vi "Set Application Error.vi"(4 "Time Stamp":timestamp, 5 "Error Name":string, 6 "Error Message":string, 7 "Error Scope":string, 8 "Error In":errorcluster, 9 "Call Chain":string[](array[string]), 10 "Log Error?":bool, 11 "Error Source":string) -> (0 "Error Out":errorcluster)   [LabVIEW 2016, in "Stream Error.lvlib" / "Application Error.lvclass"]
doc: "--\nCopyright © 2017 Composed SystemsI All rights reserved.\n\nAuthor: Jon McBee <jon.mcbee@composed.io>\n\nThis library is provided \"AS IS\" ,WITHOUT WARRANTIES OR\nCONDITIONS OF ANY KIND, either express or implied.\n\nComposed Systems -- composed.io\n\nStream 0.0.1.1\nJon McBee - Composed Systems\nCopyright (c) 2017, Composed Systems"
uses:
  <userlib>/Composed Systems/Stream/Error/Classes/Application Error/Application Error.lvclass
  <userlib>/Composed Systems/Stream/Error/Classes/Error Interface/Error Interface.lvclass
  <userlib>/Composed Systems/Stream/Error/Classes/Error Interface/Error Interface.lvclass/Error Interface.ctl
  <userlib>/Composed Systems/Stream/Log/Application Log/Log Level.ctl
  <userlib>/Composed Systems/Stream/Log/Global Application Log/Global Application Log.lvclass
  <userlib>/Composed Systems/Stream/Log/Application Log/Application Log.lvclass
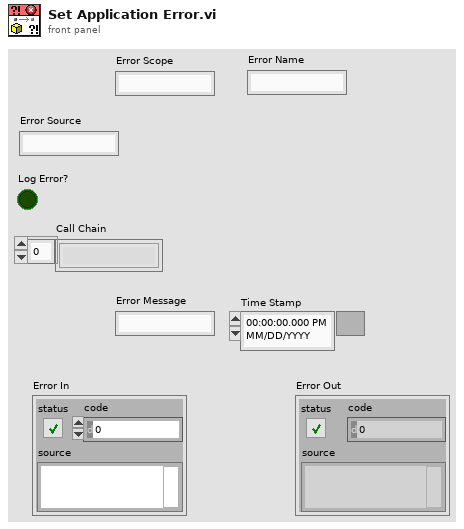
[diagram p1: front panel]
types:
  T1 = typedef "Stream Log.lvlib/Application Log.lvclass/Log Level.ctl" = enum16{"Imperative", "Major", "Minor", "Debug", "Off"}
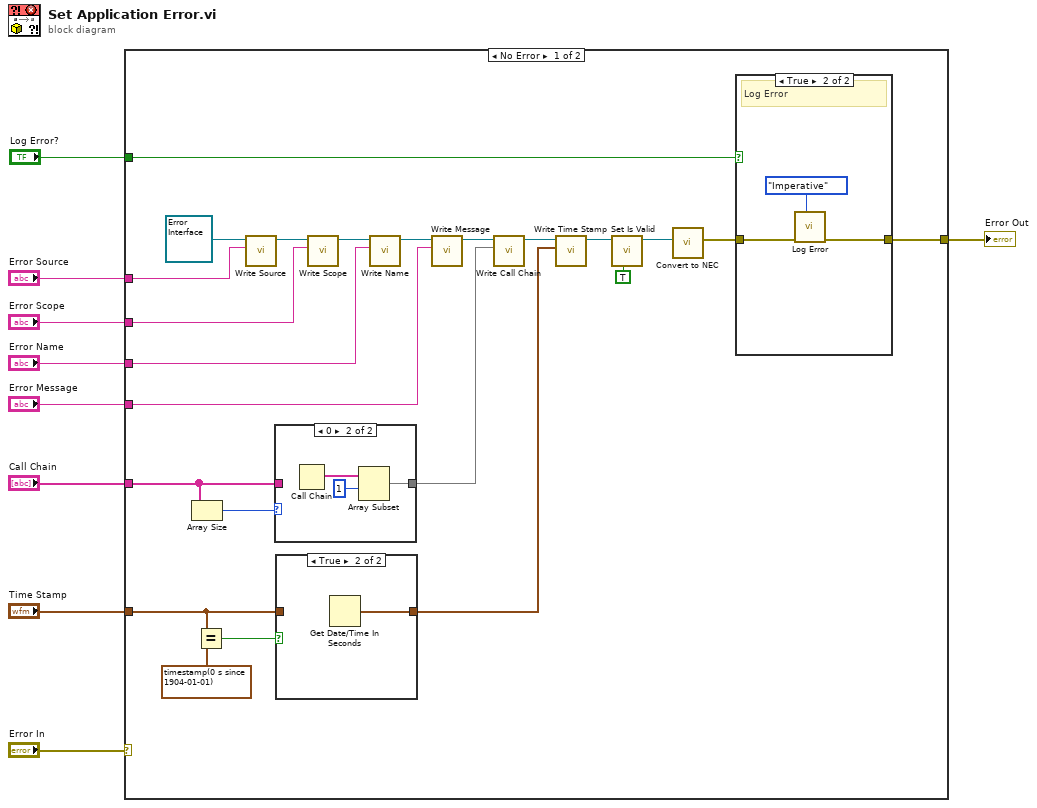
[diagram p0: block diagram]
diagram:
  n1 = case shown="No Error" "Error In" {
    selector: "Error In" -> [_ w43]
    tunnel: "Log Error?" -> [w12 _]
    tunnel: "Time Stamp" -> [w30 _]
    tunnel: "Call Chain" -> [w28 _]
    tunnel: "Error Source" -> [w26 _]
    tunnel: "Error Scope" -> [w25 _]
    tunnel: "Error Name" -> [w19 _]
    tunnel: "Error Message" -> [w18 _]
    tunnel: [w10 w43] -> w1
    frame No Error {
      n2 = Array Size(array=w28) -> (size(s)=w29:i32)
      n3 = Equal?(x=w30, y=timestamp(0 s since 1904-01-01)) -> (x = y?=w31:bool)
      n4 = call <userlib>:"Write Source.vi"("Source"=w26, "Error Interface in"=refnum<class "Error Interface.lvclass"> refnum) -> ("Error Interface out"=w24:refnum<class "Error Interface.lvclass">)  [unwired: 8 in, 1 out]
      n5 = case shown="0" w29 {
        tunnel: [w37 w38] -> w17
        tunnel: w28 -> [w37 _]
        frame Default {
        }
        frame 0 {
          n6 = Call Chain() -> (call chain=w40:string[])
          n7 = Array Subset(array=w40, index=1 ("length")) -> (w38:string[])  [unwired: 1 in]
        }
      }
      n8 = case shown="True" w31 {
        tunnel: [w41 w42] -> w16
        tunnel: w30 -> [w41 _]
        frame False {
        }
        frame True {
          n9 = Get Date/Time In Seconds() -> (seconds since 1Jan1904=w42:timestamp)
        }
      }
      n10 = call <userlib>:"Write Scope.vi"("Scope"=w25, "Error Interface in"=w24) -> ("Error Interface out"=w23:refnum<class "Error Interface.lvclass">)  [unwired: 8 in, 1 out]
      n11 = call <userlib>:"Write Name.vi"("Name"=w19, "Error Interface in"=w23) -> ("Error Interface out"=w22:refnum<class "Error Interface.lvclass">)  [unwired: 8 in, 1 out]
      n12 = call <userlib>:"Write Message.vi"("Message"=w18, "Error Interface in"=w22) -> ("Error Interface out"=w21:refnum<class "Error Interface.lvclass">)  [unwired: 8 in, 1 out]
      n13 = call <userlib>:"Write Call Chain.vi"("Call Chain"=w17, "Error Interface in"=w21) -> ("Error Interface out"=w20:refnum<class "Error Interface.lvclass">)  [unwired: 8 in, 1 out]
      n14 = call <userlib>:"Write Time Stamp.vi"("Time Stamp"=w16, "Error Interface in"=w20) -> ("Error Interface out"=w15:refnum<class "Error Interface.lvclass">)  [unwired: 8 in, 1 out]
      n15 = call <userlib>:"Set Is Valid.vi"("Valid"=TRUE, "Error Interface in"=w15) -> ("Error Interface out"=w13:refnum<class "Error Interface.lvclass">)  [unwired: 9 in]
      n16 = call <userlib>:"Convert to NEC.vi"("Error Interface in"=w13) -> ("error out"=w11:errorcluster)  [unwired: 10 in]
      n17 = case shown="True" w12 {
        tunnel: w11 -> [w33 w36]
        tunnel: [w33 w35] -> w10
        frame False {
          # "Dont Log Error"
        }
        frame True {
          # "Log Error"
          n18 = call <userlib>:"Log Error.vi"("Level"=Log_Level."Imperative", "error in (no error)"=w36) -> ("error out"=w35:errorcluster)  [unwired: 9 in]
        }
      }
    }
    frame Error {
    }
  }
  "Error Out" <- w1
